vi "sum of 'n' numbers using 'for' loop.vi"() -> ()   [LabVIEW 2024]
panel:
  out "output":dbl
  in  "Constant":dbl
  in  "Input":dbl
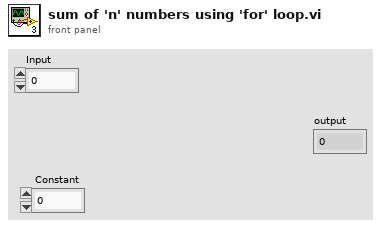
[diagram p1: front panel]
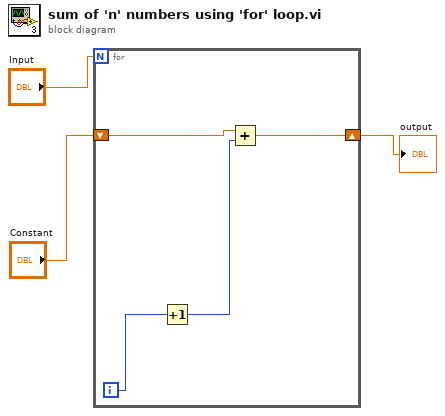
[diagram p0: block diagram]
diagram:
  n1 = for {
    N: "Input" -> [_]
    shift-right: [w5] -> w2
    shift-left: "Constant" -> [w7]
    i -> [w4]
    n2 = Increment(x=w4) -> (x+1=w6:i32)
    n3 = Add(x=w7, y=w6) -> (x+y=w5:dbl)
  }
  "output" <- w2
